vi "Error.vi"(8 "error in (no error)":errorcluster, 11 "Queue in":refnum<queue>) -> (0 "error out":errorcluster)   [LabVIEW 2019, in "AjustesPrevios.lvclass"]
uses:
  AjustesPrevios.lvclass
  Controles/MessageAjustesPrev.ctl
  Controles/EstadosAjsutesPrev.ctl
  Prueba/Prueba.lvclass
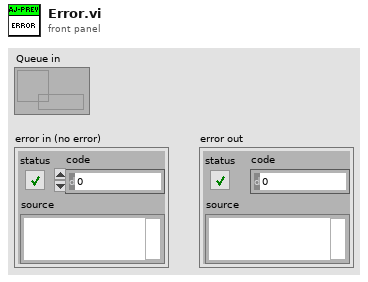
[diagram p1: front panel]
types:
  T1 = typedef "Prueba.lvclass/MessageAjustesPrev.ctl" = cluster{"Estados":T2, "Data":variant}
  T2 = typedef "Prueba.lvclass/EstadosAjsutesPrev.ctl" = enum16{"inicio", "iniciaInstrumentos", "configurarTabla", "Ajustes1", "escribeSensib", "aplicarFC", "escribir_datos_igual_patrones", "preguntar_gen", "Ajustes2", "generar", "detenerGEN", "monitorear", "guardar", "Ajustes3", "generarCAM_94", "avisoParaCAM114", "generarCAM_114", "salir", "error", "reconec_pistofono"}
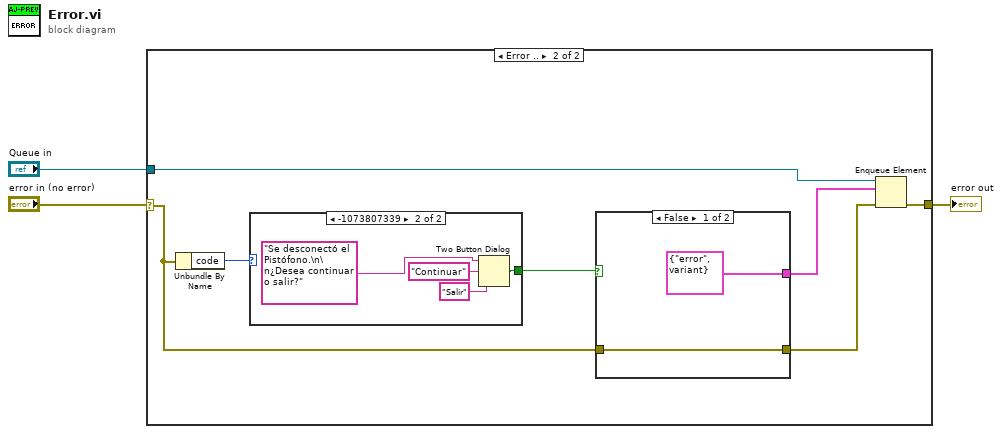
[diagram p0: block diagram]
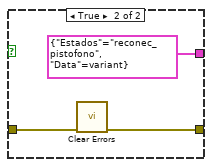
[diagram p3: hidden frame]
diagram:
  n1 = case shown="Error .." "error in (no error)" {
    selector: "error in (no error)" -> [w4 w6]
    tunnel: [w4 w11] -> w1
    tunnel: "Queue in" -> [_ w10]
    frame No Error {
    }
    frame Error {
      n2 = Unbundle By Name(w6) -> ("code"=w8:i32)
      n3 = case shown="-1073807339" w8 {
        tunnel: [_ w20] -> w7
        frame 0, Default {
        }
        frame -1073807339 {
          n4 = Two Button Dialog(message="Se desconectó el Pistófono.\n\n¿Desea continuar o salir?", 1:"Salir" ("F button name (\"Cancel\")"), 2:"Continuar" ("T button name (\"OK\")")) -> (T button?=w20:bool)
        }
      }
      n5 = case shown="False" w7 {
        tunnel: [T1 {"Estados"=enum."error", "Data"=variant} ("element") T1 {"Estados"=enum."reconec_pistofono", "Data"=variant} ("element")] -> w9
        tunnel: w6 -> [w13 w15]
        tunnel: [w13 w14] -> w5
        frame False {
        }
        frame True {
          n6 = call <vilib>:"Clear Errors.vi"("error in (no error)"=w15) -> ("error out"=w14:errorcluster)  [unwired: 5 in, 1 out]
        }
      }
      n7 = Enqueue Element(queue=w10, element=w9, error in (no error)=w5) -> (error out=w11:errorcluster)  [unwired: 1 in, 2 out]
    }
  }
  "error out" <- w1
